vi "Packet_modulate.vi"(6 "filter parameters":T3={"Alpha"=0.5, "Filter Length"=6, "TX Filter"=enum."Root Raised Cos"} {"Alpha" format="%.2f"}, 8 "error in (no error)":errorcluster, 9 "PSK Parameters":T1, 10 "IQ Sampling\nRate [S/sec]":dbl=500000.0 format="%#.6p", 11 "input bit stream":i8[](array[numeric])) -> (0 "error out":errorcluster, 2 "bits sent":i32, 3 "output complex waveform":T2 {"Y" format="%.3f"; "dt" format="%^.2e"; "t0" format="%.4f"})   [LabVIEW 2014]
uses:
  <vilib>/addons/Modulation/Analog/controls/Complex Data Waveform.ctl
  <vilib>/addons/Modulation/Analog/support/mod_Set Error Source.vi
  <vilib>/addons/Modulation/Digital/Support/Common/Validators/mod_Generate Filter Coefficients Validate.vi
  <vilib>/addons/Modulation/Digital/General/subVIs/mod_Generate Filter Coefficients.vi
  <vilib>/addons/Modulation/Digital/General/MT Generate PSK System Parameters(M).vi
  <vilib>/addons/Modulation/niDMT.lvlib
  <vilib>/addons/Modulation/niAMT.lvlib
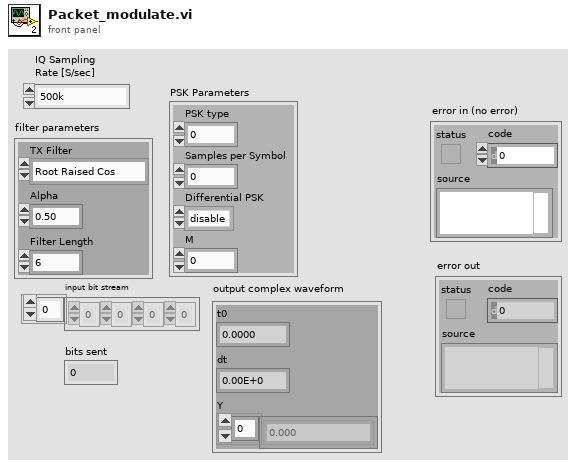
[diagram p1: front panel]
types:
  T1 = cluster{"PSK type":u16, "Samples per Symbol":i32, "Differential PSK":enum16{"disable", "enable"}, "M":i32}
  T2 = typedef "niAMT.lvlib/Complex Data Waveform.ctl" = cluster{"t0":dbl, "dt":dbl, "Y":cdb[]}
  T3 = cluster{"Alpha":dbl, "Filter Length":i32, "TX Filter":enum16{"none", "Raised Cosine", "Root Raised Cos", "Gaussian"}}
  T4 = enum16{"FSK", "PSK", "QAM", "MSK", "PAM", "ASK", "CPM"}
  T5 = enum16{"none", "Raised Cosine", "Root Raised Cos", "Gaussian"}
  T6 = cluster{"samples per symbol (16)":i32, "symbol map":cdb[], "differential PSK":enum16{"disable", "enable"}, "PSK type":u16}
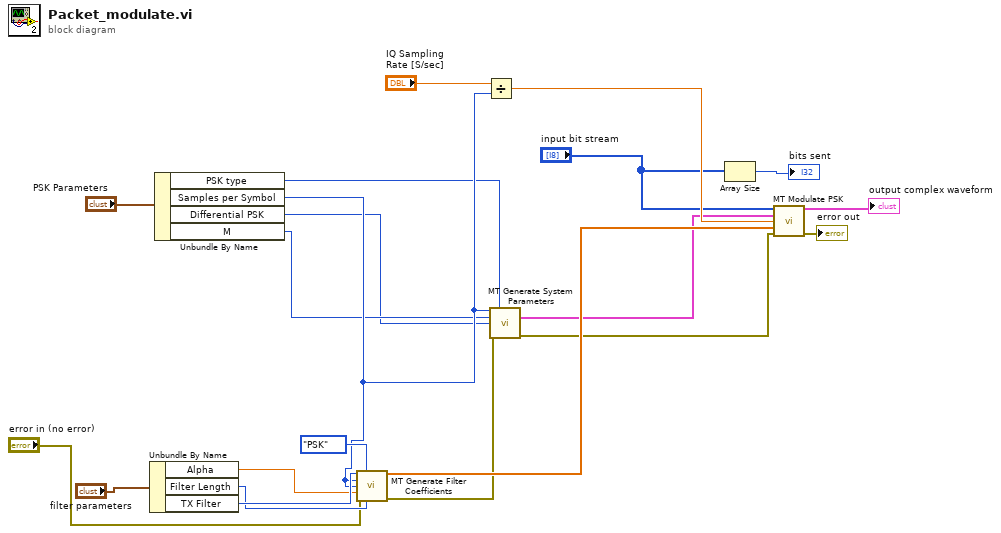
[diagram p0: block diagram]
diagram:
  n1 = Unbundle By Name("filter parameters") -> ("Alpha"=w19:dbl, "Filter Length"=w20:i32, "TX Filter"=w21:T5)
  n2 = Unbundle By Name("PSK Parameters") -> ("PSK type"=w3:u16, "Samples per Symbol"=w5:i32, "Differential PSK"=w2:enum16{"disable", "enable"}, "M"=w4:i32)
  n3 = call <vilib>:"MT Generate Filter Coefficients.vi"("pulse shaping filter (none)"=w21, "modulation type"=T4."PSK", "pulse shaping samples per symbol (16)"=w5, "matched samples per symbol (16)"=w5, "filter parameter"=w19, "error in (no error)"="error in (no error)", "filter length (symbols)"=w20) -> ("pulse shaping filter coefficients"=w16:dbl[], "error out"=w8:errorcluster)  [unwired: 6 in, 1 out]
  n4 = Divide(x="IQ Sampling\nRate [S/sec]", y=w5) -> (x/y=w15:dbl)
  n5 = call-poly <vilib>:"MT Generate System Parameters.vi"("samples per symbol (16)"=w5, "PSK type"=w3, "M-PSK (4)"=w4, "differential PSK"=w2, "error in (no error)"=w8) -> ("PSK system parameters"=w12:T6, "error out"=w7:errorcluster)  [unwired: 8 in, 1 out]
  n6 = Array Size(array="input bit stream") -> (size(s)=→"bits sent":i32)
  n7 = call <vilib>:"MT Modulate PSK.vi"("input bit stream"="input bit stream", "PSK system parameters"=w12, "symbol rate (Hz)"=w15, "pulse shaping filter coefficients"=w16, "error in (no error)"=w7) -> ("output complex waveform"=→"output complex waveform":T2, "error out"=→"error out":errorcluster)  [unwired: 8 in, 1 out]
